vi "RidgeClassifierCV.vi"(8 "error in":errorcluster) -> (0 "error out":errorcluster, 3 "out":refnum<class "RidgeClassifierCV.lvclass">)   [LabVIEW 2020]
doc: "Ridge classifier with built-in cross-validation.\n\n See glossary entry for :term:`cross-validation estimator`.\n\n By default, it performs Leave-One-Out Cross-Validation. Currently,\n only the n_features > n_samples case is handled efficiently.\n\n Read more in the :ref:`User Guide <ridge_regression>`.\n\n Parameters\n ----------\n alphas : ndarray of shape (n_alphas,), default=(0.1, 1.0, 10.0)\n Array of alpha values to try.\n Regularization strength; must be a positive float. Regularization\n improves the conditioning of the problem and reduces the variance of\n the estimates. Larger values specify stronger regularization.\n Alpha corresponds to ``1 / (2C)`` in other linear models such as\n :class:`~sklearn.linear_model.LogisticRegression` or\n :class:`~sklearn.svm.LinearSVC`.\n\n fit_intercept : bool, default=True\n Whether to calculate the intercept for this model. If set\n to false, no intercept will be used in calculations\n (i.e. data is expected to be centered).\n\n normalize : bool, default=False\n This parameter is ignored when ``fit_intercept`` is set to False.\n If True, the regressors X will be normalized before regression by\n subtracting the mean and dividing by the l2-norm.\n If you wish to standardize, please use\n :class:`~sklearn.preprocessing.StandardScaler` before calling ``fit``\n on an estimator with ``normalize=False``.\n\n scoring : string, callable, default=None\n A string (see model evaluation documentation) or\n a scorer callable object / function with signature\n ``scorer(estimator, X, y)``.\n\n cv : int, cross-validation generator or an iterable, default=None\n Determines the cross-validation splitting strategy.\n Possible inputs for cv are:\n\n - None, to use the efficient Leave-One-Out cross-validation\n - integer, to specify the number of folds.\n - :term:`CV splitter`,\n - An iterable yielding (train, test) splits as arrays of indices.\n\n Refer :ref:`User Guide <cross_validation>` for the various\n cross-validation strategies that can be used here.\n\n class_weight : dict or 'balanced', default=None\n Weights associated with classes in the form ``{class_label: weight}``.\n If not given, all classes are supposed to have weight one.\n\n The \"balanced\" mode uses the values of y to automatically adjust\n weights inversely proportional to class frequencies in the input data\n as ``n_samples / (n_classes * np.bincount(y))``\n\n store_cv_values : bool, default=False\n Flag indicating if the cross-validation values corresponding to\n each alpha should be stored in the ``cv_values_`` attribute (see\n below). This flag is only compatible with ``cv=None`` (i.e. using\n Leave-One-Out Cross-Validation).\n\n Attributes\n ----------\n cv_values_ : ndarray of shape (n_samples, n_targets, n_alphas), optional\n Cross-validation values for each alpha (if ``store_cv_values=True`` and\n ``cv=None``). After ``fit()`` has been called, this attribute will\n contain the mean squared errors (by default) or the values of the\n ``{loss,score}_func`` function (if provided in the constructor). This\n attribute exists only when ``store_cv_values`` is True.\n\n coef_ : ndarray of shape (1, n_features) or (n_targets, n_features)\n Coefficient of the features in the decision function.\n\n ``coef_`` is of shape (1, n_features) when the given problem is binary.\n\n intercept_ : float or ndarray of shape (n_targets,)\n Independent term in decision function. Set to 0.0 if\n ``fit_intercept = False``.\n\n alpha_ : float\n Estimated regularization parameter.\n\n best_score_ : float\n Score of base estimator with best alpha.\n\n .. versionadded:: 0.23\n\n classes_ : ndarray of shape (n_classes,)\n The classes labels.\n\n \nAvailable methods:\nGet Attributes\nGet Params\nSet Params"
uses:
  RidgeClassifierCV.lvclass
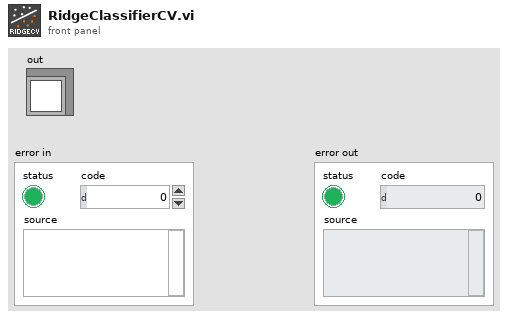
[diagram p1: front panel]
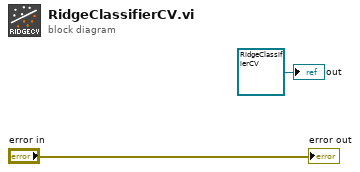
[diagram p0: block diagram]
diagram:
  "out" <- refnum<class "RidgeClassifierCV.lvclass"> refnum ("model")
  "error out" <- "error in"
